vi "Offset Widget Actions 2 Transactions.vi"(9 "Number of LBCBs":T5, 11 "Offset Widget Actions":T6) -> (2 "Transactions":T1[](array[typedef]))   [LabVIEW 2009]
uses:
  Offset Widget Actions.ctl
  Data Access Objects/Application/Number Of LBCBs.ctl
  Global Data/Transactions/Dataset Transaction Id.ctl
  Global Data/Transactions/Dataset Source.ctl
  Global Data/Transactions/Dataset Type.ctl
  Apps/Yes No Button.ctl
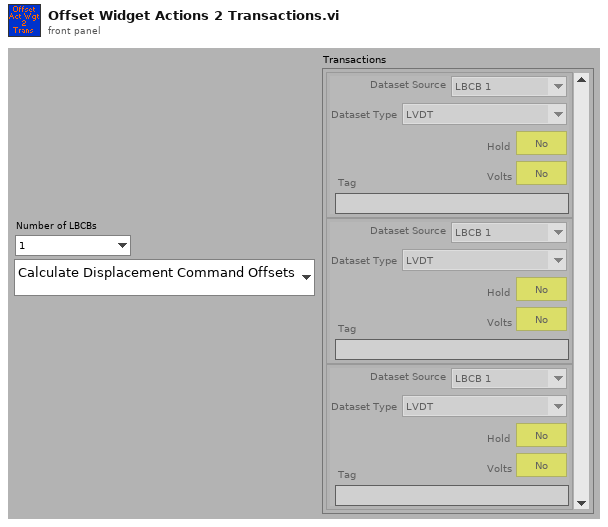
[diagram p1: front panel]
types:
  T1 = typedef "Dataset Transaction Id.ctl" = cluster{"Dataset Source":T2, "Dataset Type":T3, "Hold":T4, "Volts":T4, "Tag":string}
  T2 = typedef "Dataset Source.ctl" = enum16{"LBCB 1", "LBCB 2", "Combined", "External Sensors"}
  T3 = typedef "Dataset Type.ctl" = enum16{"LVDT", "Load Cell", "Actuator Command", "Servo Error", "Displacement Command", "Displacement", "Force"}
  T4 = typedef "Yes No Button.ctl" = bool
  T5 = typedef "Number Of LBCBs.ctl" = enum16{"1", "2"}
  T6 = typedef "Offset Widget Actions.ctl" = enum16{"Calculate Displacement Command Offsets", "Calculate Displacement Offsets", "Re-Calculate Force Offsets", "Calculate New Force Offsets", "Delete Force Offsets", "Calculate External Sensor Offsets"}
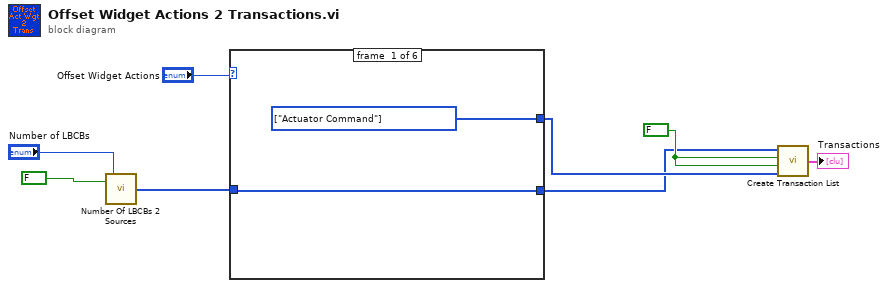
[diagram p0: block diagram]
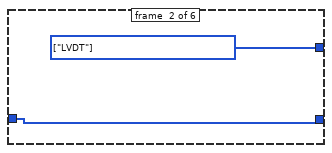
[diagram p2: hidden frame]
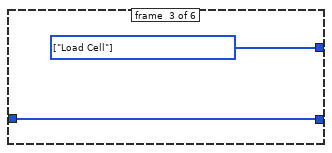
[diagram p3: hidden frame]
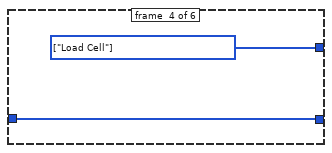
[diagram p4: hidden frame]
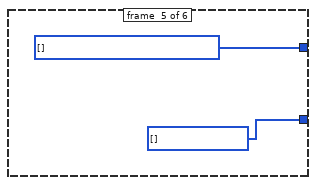
[diagram p5: hidden frame]
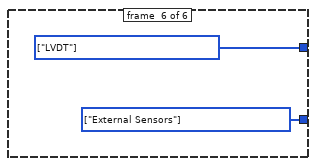
[diagram p6: hidden frame]
diagram:
  w5 = FALSE ("Include Volts")
  n1 = call "Number Of LBCBs 2 Sources.vi"("Number of LBCBs"="Number of LBCBs", "Combined LBCBs"=FALSE) -> ("Sources"=w4:T2[])
  n2 = case shown="\"Calculate Displacement Command Offsets\"" "Offset Widget Actions" {
    tunnel: [w10 w12 w14 w16 w18 w20] -> w6
    tunnel: w4 -> [w9 w11 w13 w15 _ _]
    tunnel: [w9 w11 w13 w15 w17 w19] -> w3
    frame #0 {
      w10 = T3[] [enum."Actuator Command"] items=["LVDT", "Load Cell", "Actuator Command", "Servo Error", "Displacement Command", "Displacement", "Force"] ("Types")
    }
    frame #1 {
      w12 = T3[] [enum."LVDT"] items=["LVDT", "Load Cell", "Actuator Command", "Servo Error", "Displacement Command", "Displacement", "Force"] ("Types")
    }
    frame #2 {
      w14 = T3[] [enum."Load Cell"] items=["LVDT", "Load Cell", "Actuator Command", "Servo Error", "Displacement Command", "Displacement", "Force"] ("Types")
    }
    frame #3 {
      w16 = T3[] [enum."Load Cell"] items=["LVDT", "Load Cell", "Actuator Command", "Servo Error", "Displacement Command", "Displacement", "Force"] ("Types")
    }
    frame #4 {
      w17 = T2[] [] items=["LBCB 1", "LBCB 2", "Combined", "External Sensors"] ("Sources")
      w18 = T3[] [] items=["LVDT", "Load Cell", "Actuator Command", "Servo Error", "Displacement Command", "Displacement", "Force"] ("Types")
    }
    frame #5 {
      w19 = T2[] [enum."External Sensors"] items=["LBCB 1", "LBCB 2", "Combined", "External Sensors"] ("Sources")
      w20 = T3[] [enum."LVDT"] items=["LVDT", "Load Cell", "Actuator Command", "Servo Error", "Displacement Command", "Displacement", "Force"] ("Types")
    }
  }
  n3 = call "Create Transaction List.vi"("Types"=w6, "Hold"=w5, "Volts"=w5, "Sources"=w3) -> ("Transactions"=→"Transactions":T1[])
